vi "4Pi DCM - 2D Gaussian - Fit -init.vi"(0 "Image In (DBL)":dbl[][](array[numeric]), 9 "width":dbl, 11 "Error In":errorcluster) -> (8 "Best Fit Params":T1, 15 "Error Out":errorcluster)   [LabVIEW 2016]
uses:
  4Pi Drift Monitor Controls/4Pi DCM-2D Gaussian - Best Fit Parameters.ctl
  <vilib>/gmath/NumericalOptimization/Nonlinear Curve Fit LM bound.vi
  <vilib>/gmath/NI_Gmath.lvlib
panel:
  out "MSE":dbl
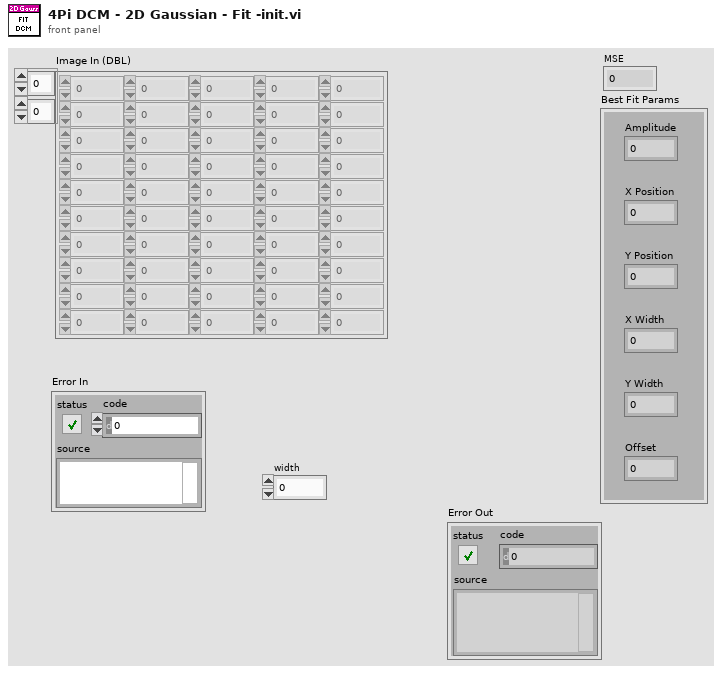
[diagram p1: front panel]
types:
  T1 = typedef "4Pi DCM-2D Gaussian - Best Fit Parameters.ctl" = cluster{"Amplitude":dbl, "X Position":dbl, "Y Position":dbl, "X Width":dbl, "Y Width":dbl, "Offset":dbl}
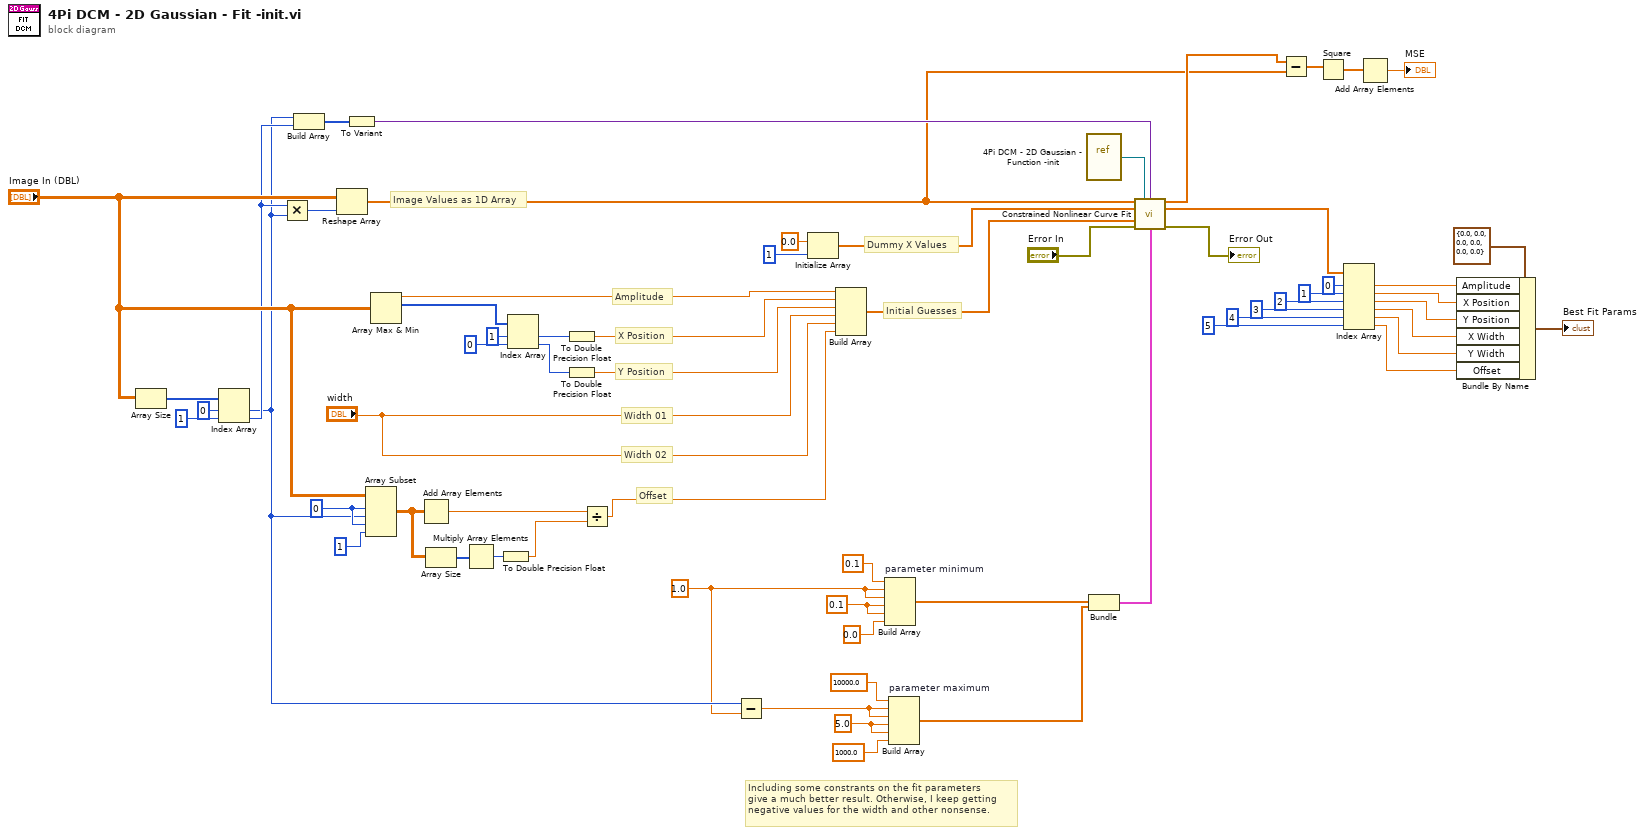
[diagram p0: block diagram]
diagram:
  w8 = 5.0 ("element")
  w11 = 0.1 ("element")
  w5 = 1.0 ("element")
  w13 = 0 ("index")
  # "Including some constrants on the fit parameters\ngive a much better result. Otherwise, I keep getting\nnegative values for the width and other nonsense."
  # "Dummy X Values"
  # "Image Values as 1D Array"
  # "Initial Guesses"
  # "Width 02"
  # "Width 01"
  # "Y Position"
  # "X Position"
  # "Offset"
  # "Amplitude"
  n1 = Array Size(array="Image In (DBL)") -> (size(s)=w54:i32[])
  n2 = Index Array(array=w54, index #1=0 ("index"), index #2=1 ("index")) -> (element #1=w6:i32, element #2=w21:i32)
  n3 = Multiply(x=w21, y=w6) -> (x*y=w53:i32)
  n4 = Build Array(w6, w21) -> (w49:i32[])
  n5 = Reshape Array("Image In (DBL)", w53) -> (w27:dbl[])
  n6 = To Variant(anything=w49) -> (Variant=w48:variant)
  n7 = Array Subset(array="Image In (DBL)", index (row)=w13, length (row)=w6, index (col)=w13, length (col)=1 ("length")) -> (w20:dbl[][])
  n8 = Array Max & Min(array="Image In (DBL)") -> (max value=w30:dbl, max index (indices)=w63:i32[])  [unwired: 2 out]
  n9 = Add Array Elements(numeric array=w20) -> (sum=w18:dbl)
  n10 = Array Size(array=w20) -> (size(s)=w19:i32[])
  n11 = Multiply Array Elements(1:w19) -> (0:w17:i32)
  n12 = To Double Precision Float(number=w17) -> (double precision float=w16:dbl)
  n13 = Index Array(array=w63, index #1=1 ("index"), index #2=0 ("index")) -> (element #1=w60:i32, element #2=w58:i32)
  n14 = To Double Precision Float(number=w60) -> (double precision float=w59:dbl)
  n15 = To Double Precision Float(number=w58) -> (double precision float=w57:dbl)
  n16 = Divide(x=w18, y=w16) -> (x/y=w15:dbl)
  n17 = Subtract(x=w6, y=w5) -> (x-y=w4:dbl)
  n18 = Initialize Array(0.0 ("element"), 1 ("dimension size")) -> (w51:dbl[])
  n19 = Build Array(w30, w59, w57, "width", "width", w15) -> (w50:dbl[])
  n20 = Build Array "parameter minimum"(0.1 ("element"), w5, w5, w11, w11, 0.0 ("element")) -> (w3:dbl[])
  n21 = Build Array "parameter maximum"(10000.0 ("element"), w4, w4, w8, w8, 1000.0 ("element")) -> (w2:dbl[])
  n22 = vi-ref "4Pi DCM - 2D Gaussian - Function -init.vi"() -> (w64:refnum<vi>)
  n23 = Bundle(w3, w2) -> (w1:cluster{dbl[], dbl[]})  [unwired: 1 in]
  n24 = call-poly <vilib>:"Constrained Nonlinear Curve Fit.vi"("Y"=w27, "f(x,a)"=w64, "data"=w48, "X"=w51, "initial parameters"=w50, "error in (no error)"="Error In", "parameter bounds"=w1) -> ("best nonlinear fit"=w28:dbl[], "best fit parameters"=w46:dbl[], "error out"=→"Error Out":errorcluster)  [unwired: 3 in, 3 out]
  n25 = Subtract(x=w28, y=w27) -> (x-y=w26:dbl[])
  n26 = Square(x=w26) -> (x^2=w25:dbl[])
  n27 = Index Array(array=w46, index #1=0 ("index"), index #2=1 ("index"), index #3=2 ("index"), index #4=3 ("index"), index #5=4 ("index"), index #6=5 ("index")) -> (element #1=w45:dbl, element #2=w44:dbl, element #3=w43:dbl, element #4=w42:dbl, element #5=w41:dbl, element #6=w40:dbl)
  n28 = Add Array Elements(numeric array=w25) -> (sum=→"MSE":dbl)
  n29 = Bundle By Name(cluster=T1 {"Amplitude"=0.0, "X Position"=0.0, "Y Position"=0.0, "X Width"=0.0, "Y Width"=0.0, "Offset"=0.0} ("Best Fit Parameters"), "Amplitude"=w45, "X Position"=w44, "Y Position"=w43, "X Width"=w42, "Y Width"=w41, "Offset"=w40) -> (→"Best Fit Params":T1)
